vi "Set DDS Burst Delay Ns.vi"(10 "ns":cluster{}, 11 "channel_index":u8) -> ()   [LabVIEW 2021, in "vmmso.lvlib"]
doc: "DLL_API void WINAPI SetDDSBurstDelayNs(unsigned char channel_index, unsigned long long int ns);"
uses:
  vmmso.lvlib
  vmmso.dll
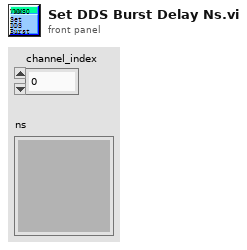
[diagram p1: front panel]
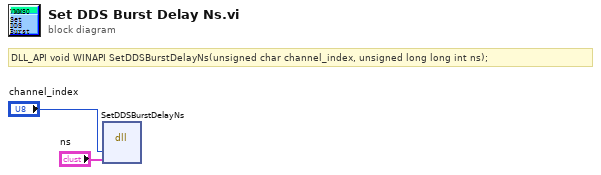
[diagram p0: block diagram]
diagram:
  # "DLL_API void WINAPI SetDDSBurstDelayNs(unsigned char channel_index, unsigned long long int ns);"
  n1 = dll-call lib="D:/labviewdemo/LabviewDemo 21/vmmso/vmmso.*" fn="SetDDSBurstDelayNs"("channel_index"="channel_index", "ns"="ns") -> ()  [unwired: 6 in, 2 out]
